vi "Scrub.vi"(8 "error in":errorcluster, 10 "Input String":string, 11 "Regex Scrubber in":refnum<class "Regex Scrubber.lvclass">) -> (0 "error out":errorcluster, 2 "Scrubbed String":string, 3 "Regex Scrubber out":refnum<class "Regex Scrubber.lvclass">)   [LabVIEW 2020, in "Approval Tests.lvlib" / "Regex Scrubber.lvclass"]
uses:
  Regex Scrubber.lvclass
  Regex Scrubber.lvclass/Regex Scrubber.ctl
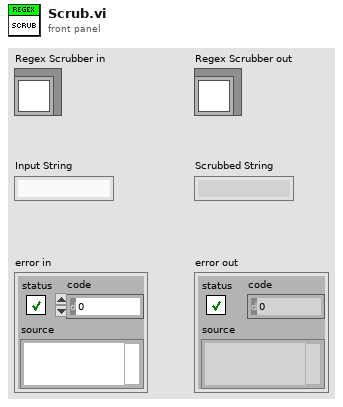
[diagram p1: front panel]
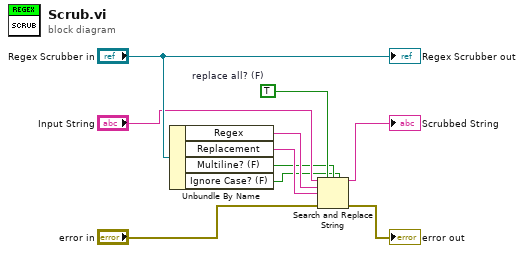
[diagram p0: block diagram]
diagram:
  w3 = TRUE  # replace all? (F)
  n1 = Unbundle By Name("Regex Scrubber in") -> ("Regex"=w5:string, "Replacement"=w4:string, "Multiline? (F)"=w2:bool, "Ignore Case? (F)"=w1:bool)
  n2 = Search and Replace String(replace all?=w3, case sensitive?=w2, multiline?=w1, input string="Input String", search string=w5, replace string=w4, error in="error in") -> (result string=→"Scrubbed String":string, error out=→"error out":errorcluster)  [unwired: 1 in, 2 out]
  "Regex Scrubber out" <- "Regex Scrubber in"
